vi "PleaseWait.vi"(1 "Current Test 2":string) -> ()   [LabVIEW 2024]
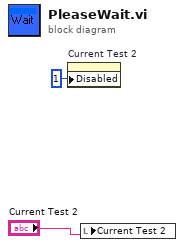
[diagram p0: block diagram]
diagram:
  n1 = property on="Current Test 2" class="Str"("Disabled"=u8 1) -> ()  [unwired: 2 in, 2 out]
  n2 = local write "Current Test 2"("Current Test 2") -> ()
